vi "Renishaw-XL80_GetPressure.vi"(8 "error in (no error)":errorcluster, 11 "Renishaw-XL80_EMU in":refnum<class "Renishaw-XL80_EMU.lvclass">) -> (0 "error out":errorcluster, 1 "pStatus":i32(ring) items=["SENSOR_OK"=0, "SENSOR_BAD_READING"=1, "SENSOR_FAILED"=2, "SENSOR_NOT_CONNECTED"=4], 2 "GetPressure":dbl, 3 "Renishaw-XL80_EMU out":refnum<class "Renishaw-XL80_EMU.lvclass">)   [LabVIEW 2024, in "Renishaw-XL80_EMU.lvclass"]
doc: "This method gets the latest reading (in Pa) and status from the air pressure sensor.\n\nDefinition\nHRESULTGetPressure( [out] SENSOR_STATUS_CODES *pStatus, [out, retval] double *pVal);\nParameters\npStatus\nA variable that will be set to one of the SENSOR_STATUS_CODES.\n\npVal\nA variable that will be set to the air pressure reading (in Pa).\n\nComments\nIf the client has not connected to the DX10 then the default value (101325 Pa) will be returned and the status will be set to SENSOR_NOT_CONNECTED.\n\nIf the client connected to a DX10 and it subsequently stopped responding, or the EC10 stopped responding then the last values obtained from the EC10 will be returned i.e. the status will not be modified. It is important therefore to monitor both the DX10Status and EC10Status. This is easily done using the _RenishawDX10Events interface.\n\n\nIf the sensor status is SENSOR_NOT_CONNECTED or SENSOR_BAD_READING, then pVal will be set to the last known valid reading.\n\nThe property will normally return an HRESULT of S_OK. However, it will return E_POINTER if the client supplies a null pointer for either pVal or pStatus."
uses:
  Renishaw-XL80_EMU.lvclass
  <vilib>/numeric/Random Number (Range) DBL.vi
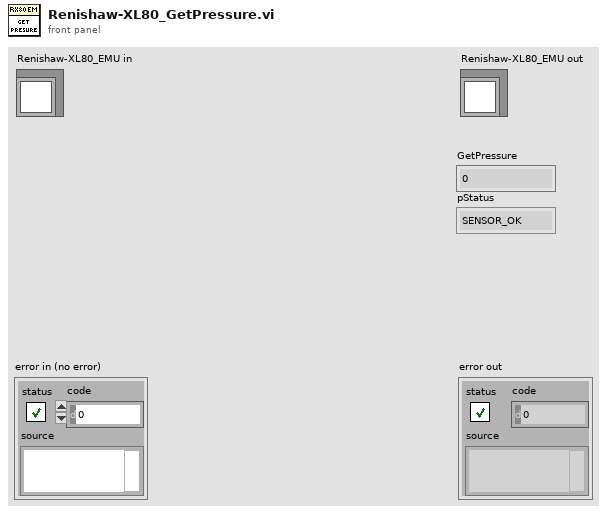
[diagram p1: front panel]
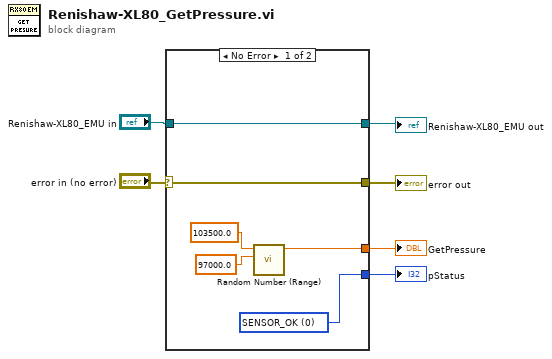
[diagram p0: block diagram]
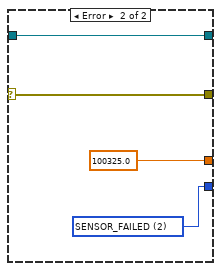
[diagram p2: hidden frame]
diagram:
  n1 = case shown="No Error" "error in (no error)" {
    selector: "error in (no error)" -> [w11 w15]
    tunnel: [w12 w16] -> w6
    tunnel: "Renishaw-XL80_EMU in" -> [w12 w16]
    tunnel: [w11 w15] -> w1
    tunnel: [w8 100325.0 ("GetAirTemp")] -> w4
    tunnel: [w7 w13] -> w3
    frame No Error {
      w7 = 0 items=["SENSOR_OK"=0, "SENSOR_BAD_READING"=1, "SENSOR_FAILED"=2, "SENSOR_NOT_CONNECTED"=4] ("pStatus")
      n2 = call-poly <vilib>:"Random Number (Range).vi"("lower bound (0)"=97000.0, "upper bound (100)"=103500.0) -> ("number"=w8:dbl)  [unwired: 9 in]
    }
    frame Error {
      w13 = 2 items=["SENSOR_OK"=0, "SENSOR_BAD_READING"=1, "SENSOR_FAILED"=2, "SENSOR_NOT_CONNECTED"=4] ("pStatus")
    }
  }
  "error out" <- w1
  "Renishaw-XL80_EMU out" <- w6
  "GetPressure" <- w4
  "pStatus" <- w3
